vi "test_rig_main.vi"(10 "Pressure Controls":T1={"Atm Press"=0.0, "Des P drop"=0.0, "Phi"=0.0, "PID gains"={"proportional gain (Kc)"=3.0, "integral time (Ti, min)"=0.0003, "derivative time (Td, min)"=-0.0001}, "output range"={"output high"=400.0, "output low"=0.0003}, "Run Mode"=enum."Non pre-mixed"} {"output range"."output low" format="%.2f"; "output range"."output high" format="%.2f"; "PID gains"."derivative time (Td, min)" format="%.6f"; "PID gains"."integral time (Ti, min)" format="%.5f"; "PID gains"."proportional gain (Kc)" format="%.3f"; "Phi" scale=0.0..1.5; "Des P drop" scale=0.0..6.0}) -> (2 "Pressure Indicators":T3 {"Measured Pressure (psi abs)" scale=0.0..6.0})   [LabVIEW 2013]
doc: "This is the main VI for the test rig program. It allows the user to control fuel flow to burners, and move\nthe three-axis table."
uses:
  Controls/pressure_control_cluster.ctl
  Controls/run_mode_enum.ctl
  Controls/pressure_indicator_cluster.ctl
  Controls/enable_control_cluster.ctl
  Controls/manual_feed_control_cluster.ctl
  Controls/axis_indicator_cluster.ctl
  Controls/auto_feed_control_cluster.ctl
  <vilib>/MotionAssistant/MotionAssistant.llb/Move Constraints.ctl
  <vilib>/MotionAssistant/MotionAssistant.llb/Velocity Profile Type Enum.ctl
  <vilib>/MotionAssistant/MotionAssistant.llb/Straight Line Move Properties.ctl
  <vilib>/MotionAssistant/MotionAssistant.llb/Straight Line Dimension Enum.ctl
  <vilib>/MotionAssistant/MotionAssistant.llb/Straight Line Move Mode Enum.ctl
  <vilib>/MotionAssistant/MotionAssistant.llb/Coordinate Point.ctl
  <vilib>/MotionAssistant/MotionAssistant.llb/Profile Calculation Constraint.ctl
  <vilib>/MotionAssistant/MotionAssistant.llb/Array Constraints Spec Type Enum.ctl
  <vilib>/MotionAssistant/MotionAssistant.llb/Move Profile Enum.ctl
  Controls/PWM_data_cluster.ctl
  Controls/table_axis_enum.ctl
  Controls/PWM_state_enum.ctl
  <vilib>/DAQmx/read.llb/DAQmx Read (Analog DBL 1Chan 1Samp).vi
  <vilib>/DAQmx/write.llb/DAQmx Write (Digital Bool 1Line 1Point).vi
  <vilib>/MotionAssistant/MotionAssistant.llb/Open Straight Line Move Handle.vi
  <vilib>/MotionAssistant/MotionAssistant.llb/Close Straight Line Move Handle.vi
  <vilib>/DAQmx/miscellaneous.llb/DAQmx Fill In Error Info.vi
  <vilib>/MotionAssistant/MotionAssistant.llb/Set Straight Line Move Properties.vi
  <vilib>/MotionAssistant/MotionAssistant.llb/Get Straight Line Move Profile.vi
panel:
  in  "stop":bool
  in  "Control Tabs":enum32{"Master Control", "Table Control"}(tab)
  in  "Enabling Controls":T4 {"Number of Images" min=0 step=1}
  out "UV Image":T5(plugin-control)
  in  "Auto Fd. Ctrl.":T6 caption="Auto Feed Control"
  out "Axis Inds.":T7 caption="Axis Indicators"
  in  "Man. Fd. Ctrl.":T8 caption="Manual Feed Control"
  in  "Move Constraints":T9={"Velocity Profile Type"=enum."S Curve", "Max Velocity"=2.0, "Max Acceleration"=1.0, "Max Deceleration"=1.0, "Max Jerk"=2.0, "Initial Velocity"=0.0, "Final Velocity"=0.0} {"Final Velocity" format="%#.6g"; "Initial Velocity" format="%#.6g"; "Max Jerk" format="%#.6g"; "Max Deceleration" format="%#.6g"; "Max Acceleration" format="%#.6g"; "Max Velocity" format="%#.6g"}
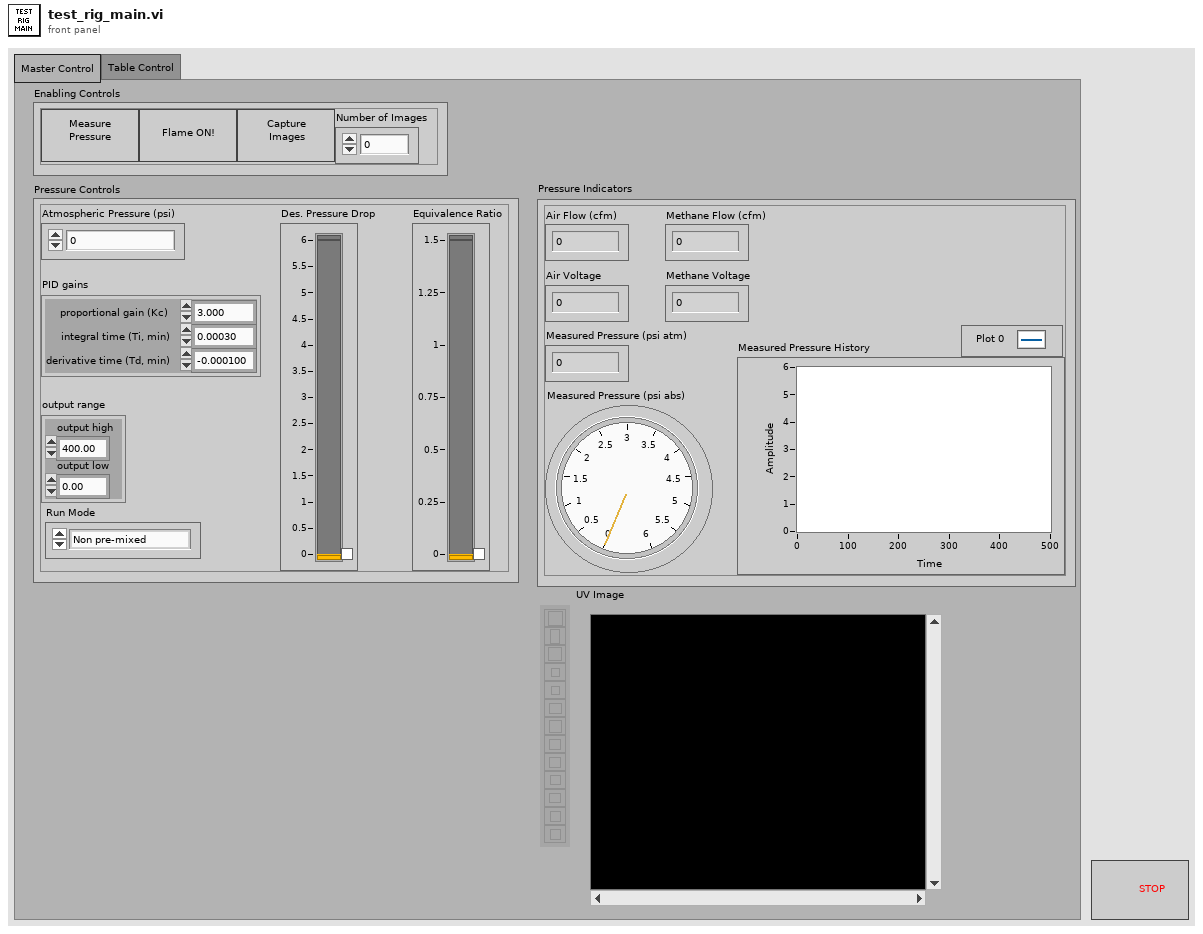
[diagram p1: front panel]
types:
  T1 = typedef "pressure_control_cluster.ctl" = cluster{"Atm Press":dbl, "Des P drop":dbl, "Phi":dbl, "PID gains":cluster{"proportional gain (Kc)":dbl, "integral time (Ti, min)":dbl, "derivative time (Td, min)":dbl}, "output range":cluster{"output high":dbl, "output low":dbl}, "Run Mode":T2}
  T2 = typedef "run_mode_enum.ctl" = enum16{"Non pre-mixed", "Pre-mixed"}
  T3 = typedef "pressure_indicator_cluster.ctl" = cluster{"Air Flow (cfm)":dbl, "Methane Flow (cfm)":dbl, "Air Voltage":dbl, "Methane Voltage":dbl, "Measured Pressure (psi atm)":dbl, "Measured Pressure (psi abs) ":dbl, "Measured Pressure History":dbl}
  T4 = typedef "enable_control_cluster.ctl" = cluster{"meas pressure":bool, "enable fuel":bool, "capture":bool, "Number of Images":i32}
  T5 = typedef "IMAQ Image.ctl" = refnum<image>
  T6 = typedef "auto_feed_control_cluster.ctl" = cluster{"Feed Rate (in/s)":dbl, "X Command (in)":dbl, "Y Command (in)":dbl, "Z Command (in)":dbl, "feed to pos":bool}
  T7 = typedef "axis_indicator_cluster.ctl" = cluster{"X Position (in)":dbl, "Y Position (in)":dbl, "Z Position (in)":dbl, "X Moving":bool, "Y Moving":bool, "Z Moving":bool, "Speed (in/s)":dbl}
  T8 = typedef "manual_feed_control_cluster.ctl" = cluster{"move -Y":bool, "move +Y":bool, "move -X":bool, "move +X":bool, "move +Z":bool, "move -Z":bool}
  T9 = typedef "Move Constraints.ctl" = cluster{"Velocity Profile Type":T10, "Max Velocity":dbl, "Max Acceleration":dbl, "Max Deceleration":dbl, "Max Jerk":dbl, "Initial Velocity":dbl, "Final Velocity":dbl}
  T10 = typedef "Velocity Profile Type Enum.ctl" = enum32{"Trapezoidal", "S Curve"}
  T11 = typedef "Straight Line Move Properties.ctl" = cluster{"Dimension":T12, "Move Mode":T13, "Position Mode - End Point":T14, "Velocity Mode - Travel Time (sec)":dbl}
  T12 = typedef "Straight Line Dimension Enum.ctl" = enum16{"1-Dimension", "2-Dimension", "3-Dimension"}
  T13 = typedef "Straight Line Move Mode Enum.ctl" = enum32{" Position Mode", "Velocity Mode"}
  T14 = typedef "Coordinate Point.ctl" = cluster{"X":dbl, "Y":dbl, "Z":dbl}
  T15 = cluster{"Straight Line Move Properties":T11, "Start Point":T14}
  T16 = typedef "Straight Line Move Handle.ctl" = cluster{"Straight Line Move Enum":T17, "Move Handle":i32}
  T17 = typedef "Straight Line Move Enum.ctl" = enum16{"Straight Line Move"}
  T18 = typedef "PWM_data_cluster.ctl" = cluster{"frequency":dbl, "Duty Cycle (%)":dbl, "Axis Enum":T19, "Function Enum":T20}
  T19 = typedef "table_axis_enum.ctl" = enum16{"X-axis", "Y-axis", "Z-axis", "W-axis"}
  T20 = typedef "PWM_state_enum.ctl" = enum16{"Initialize", "SetAxisSpeed", "StopAxis", "StopAll", "Shutdown"}
  T21 = typedef "Move Profile Enum.ctl" = enum16{"Velocity Profile", "Acceleration Profile", "Position Profile"}
  T22 = typedef "Profile Calculation Constraint.ctl" = cluster{"Constraint Type":T23, "Constraint Value":dbl}
  T23 = typedef "Array Constraints Spec Type Enum.ctl" = enum16{"Array Size", "Sampling Time"}
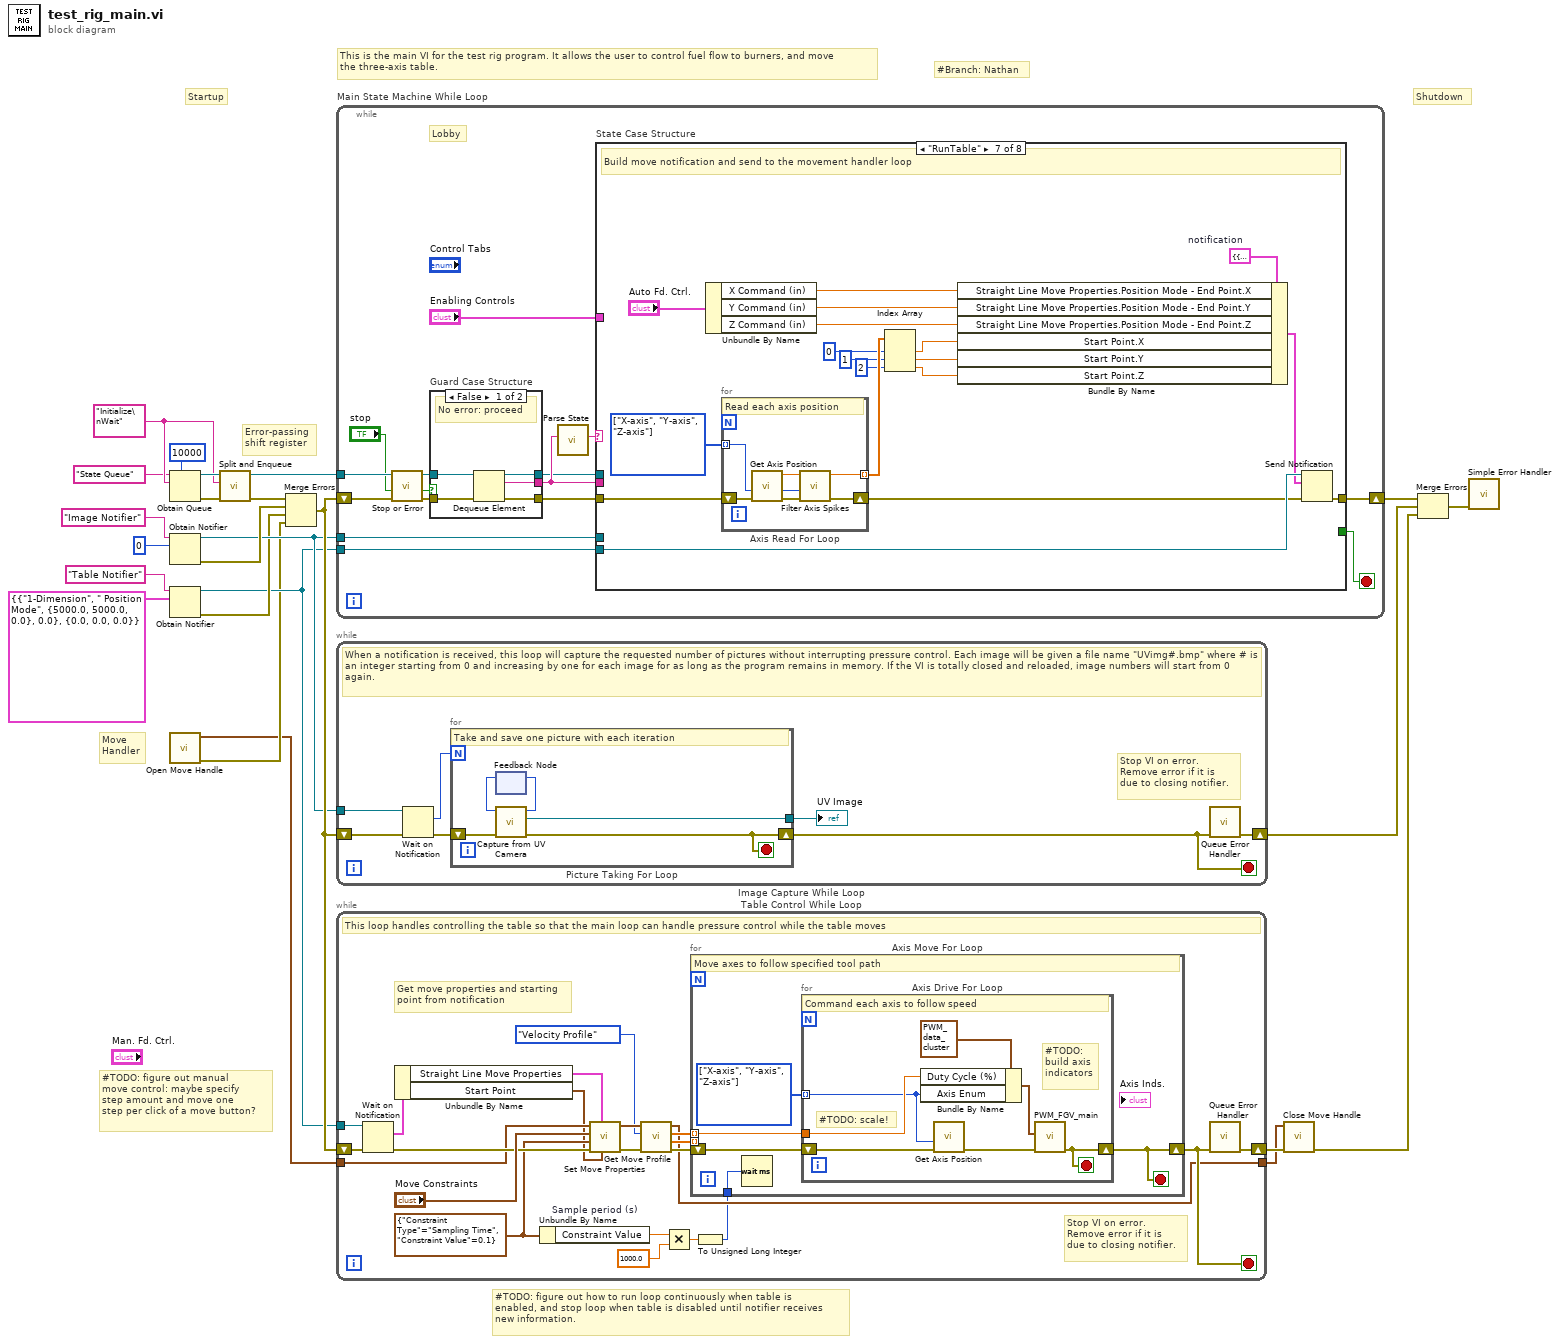
[diagram p0: block diagram]
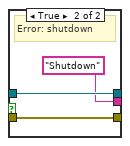
[diagram p2: hidden frame]
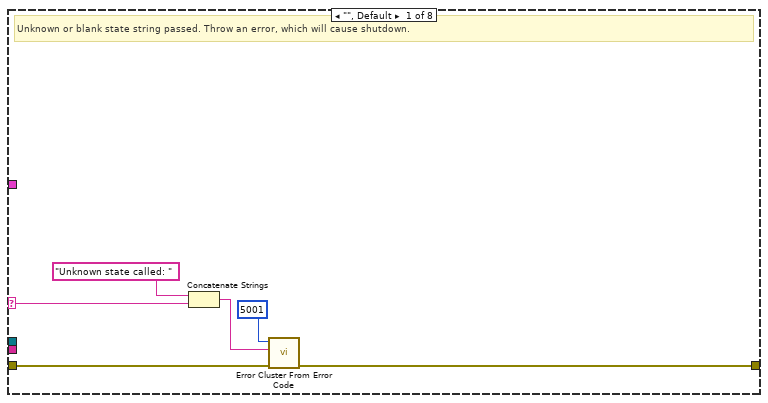
[diagram p3: hidden frame]
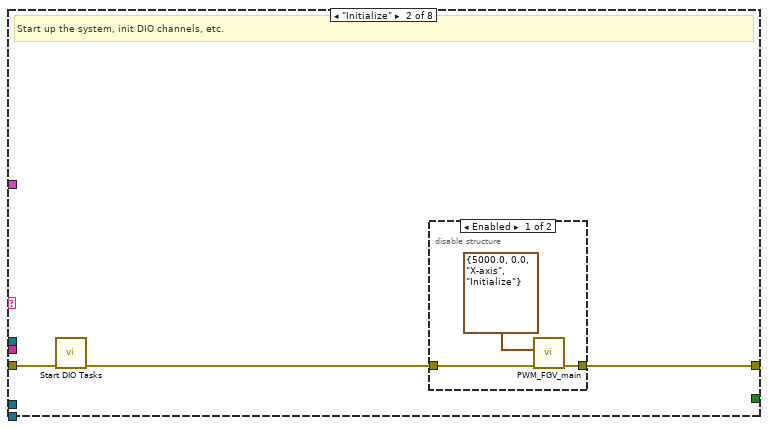
[diagram p4: hidden frame]
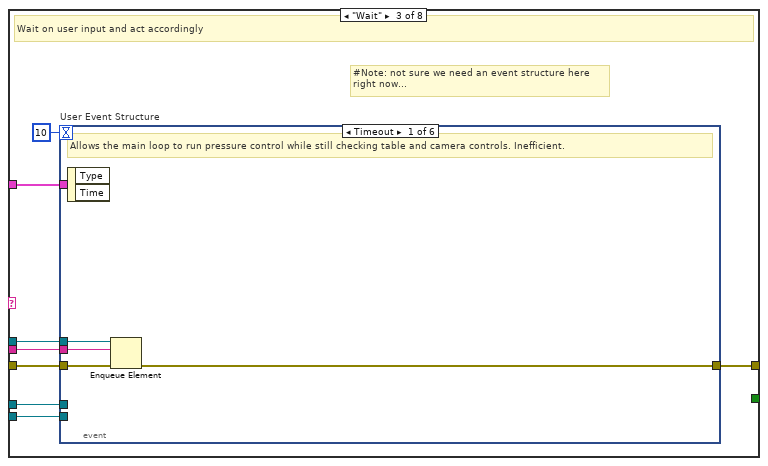
[diagram p6: hidden frame]
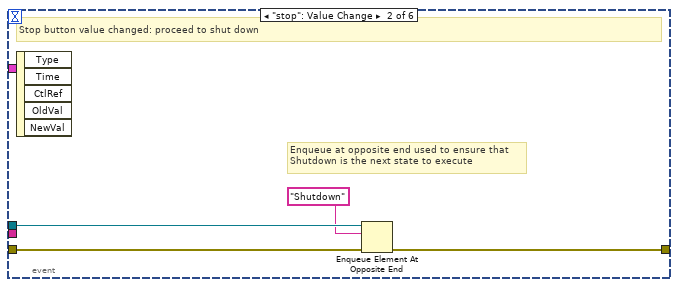
[diagram p7: hidden frame]
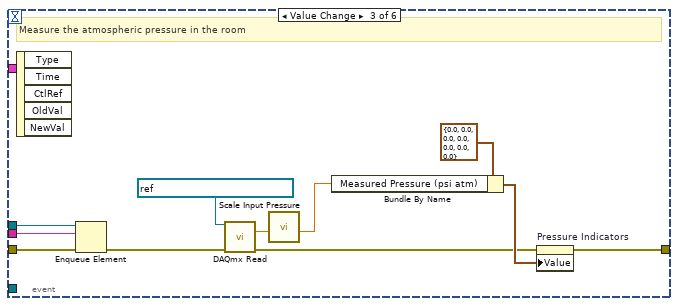
[diagram p8: hidden frame]
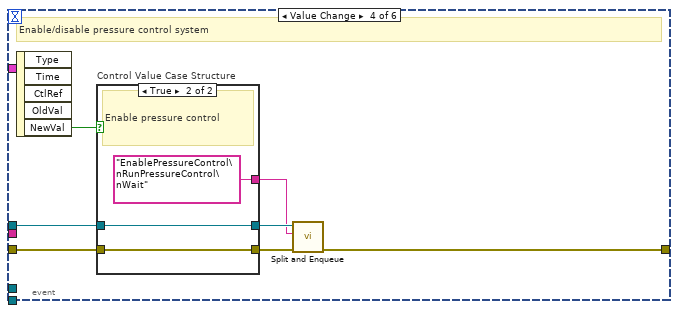
[diagram p9: hidden frame]
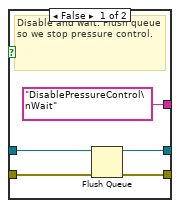
[diagram p10: hidden frame]
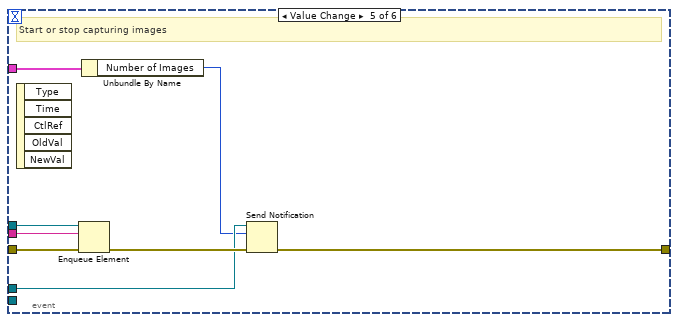
[diagram p11: hidden frame]
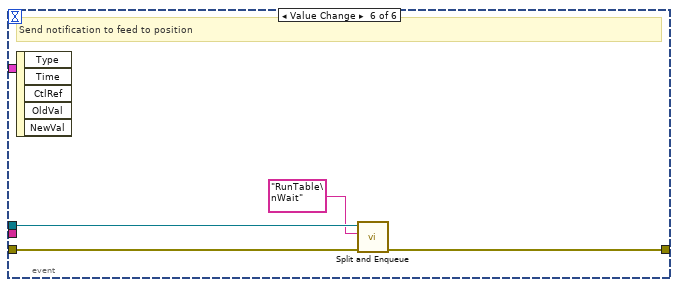
[diagram p12: hidden frame]
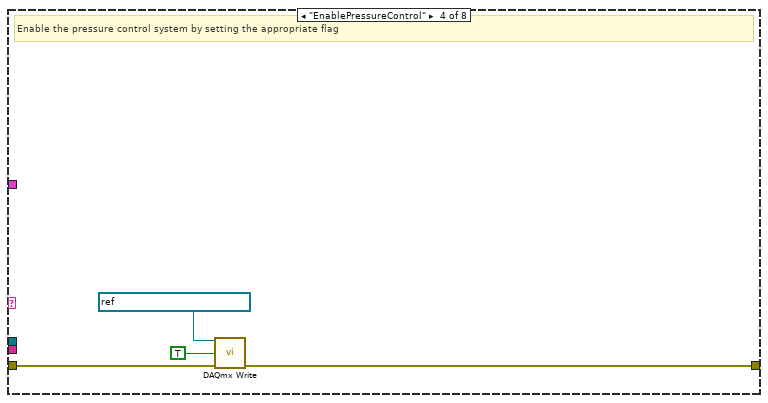
[diagram p13: hidden frame]
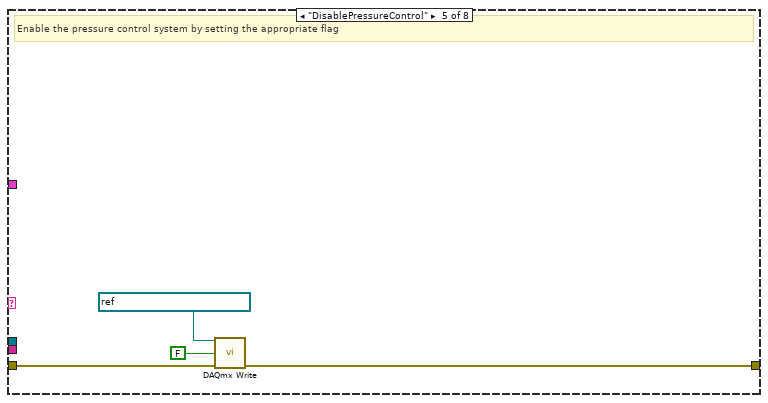
[diagram p14: hidden frame]
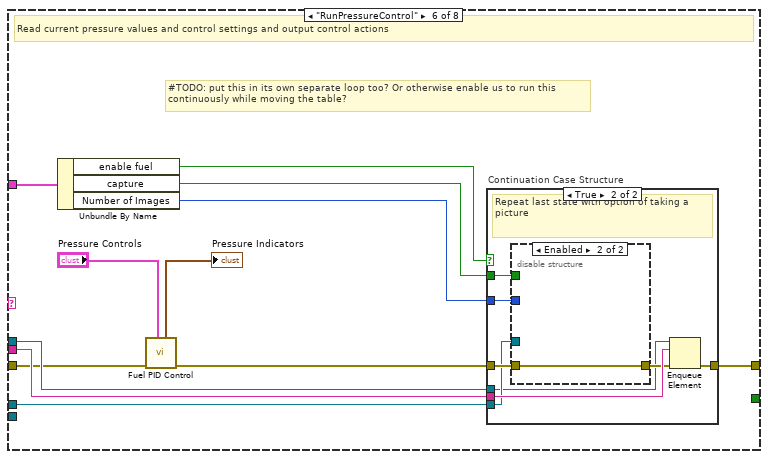
[diagram p15: hidden frame]
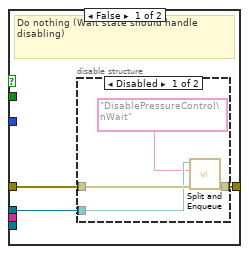
[diagram p16: hidden frame]
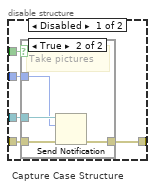
[diagram p18: hidden frame]
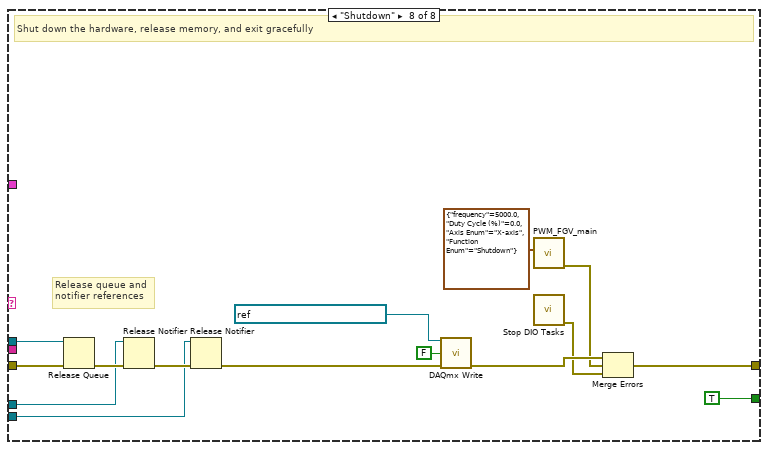
[diagram p20: hidden frame]
diagram:
  w20 = "Initialize\nWait"
  # "#Branch: Nathan"
  # "#TODO: figure out manual\nmove control: maybe specify\nstep amount and move one\nstep per click of a move button?"
  # "Move\nHandler"
  # "#TODO: figure out how to run loop continuously when table is\nenabled, and stop loop when table is disabled until notifier receives\nnew information."
  # "Shutdown"
  # "Startup"
  # "Error-passing\nshift register"
  # "This is the main VI for the test rig program. It allows the user to control fuel flow to burners, and move\nthe three-axis table."
  n1 = Obtain Queue(max queue size (-1, unlimited)=10000, name (unnamed)="State Queue", element data type=w20) -> (queue out=w22:refnum<queue>, error out=w23:errorcluster)  [unwired: 2 in, 1 out]
  n2 = Obtain Notifier(name (unnamed)="Image Notifier", notification data type=0) -> (notifier out=w10:refnum<notifier>, error out=w13:errorcluster)  [unwired: 2 in, 1 out]
  n3 = Obtain Notifier(name (unnamed)="Table Notifier", notification data type=T15 {"Straight Line Move Properties"={"Dimension"=enum."1-Dimension", "Move Mode"=enum." Position Mode", "Position Mode - End Point"={"X"=5000.0, "Y"=5000.0, "Z"=0.0}, "Velocity Mode - Travel Time (sec)"=0.0}, "Start Point"={"X"=0.0, "Y"=0.0, "Z"=0.0}}) -> (notifier out=w7:refnum<notifier>, error out=w9:errorcluster)  [unwired: 2 in, 1 out]
  n4 = call-poly <vilib>:"Open Move Handle.vi"() -> ("error out"=w6:errorcluster, "Straight Line Move Handle"=w5:T16)  [unwired: 9 in]
  n5 = call "Split and Enqueue.vi"("error in (no error)"=w23, "Input String"=w20, "queue in"=w22) -> ("error out"=w14:errorcluster, "queue out"=w21:refnum<queue>)  [unwired: 7 in]
  n6 = Merge Errors(w14, w13, w9, w6) -> (w11:errorcluster)
  n7 = while "Main State Machine While Loop" {
    tunnel: w21 -> [w38]
    shift-right: [w29] -> w12
    shift-left: w11 -> [w37]
    tunnel: w10 -> [w26]
    tunnel: w7 -> [w25]
    stop <- w28 stop-if-true
    # "Lobby"
    n8 = call "Stop or Error.vi"("Error In"=w37, "Stop Button"="stop") -> ("Error Out"=w36:errorcluster, "Stop or Error?"=w35:bool)  [unwired: 8 in]
    n9 = case "Guard Case Structure" shown="False" w35 {
      tunnel: w38 -> [w41 w45]
      tunnel: w36 -> [w43 w46]
      tunnel: [w42 w46] -> w30
      tunnel: [w40 w45] -> w31
      tunnel: [w39 "Shutdown"] -> w33
      frame False {
        # "No error: proceed"
        n10 = Dequeue Element(queue=w41, error in (no error)=w43) -> (queue out=w40:refnum<queue>, element=w39:string, error out=w42:errorcluster)  [unwired: 1 in, 1 out]
      }
      frame True {
        # "Error: shutdown"
      }
    }
    n11 = call "Parse State.vi"("String with Args"=w33) -> ("State"=w32:string)  [unwired: 10 in]
    n12 = case "State Case Structure" shown="\"RunTable\"" w32 {
      selector: w32 -> [w49 _ _ _ _ _ _ _]
      tunnel: w33 -> [_ _ w64 _ _ w131 _ _]
      tunnel: w31 -> [_ _ w65 _ _ w132 _ w199]
      tunnel: w30 -> [w52 w55 w67 w117 w119 w128 w178 w200]
      tunnel: [w51 w54 w66 w116 w118 w133 w173 w197] -> w29
      tunnel: [_ _ _ _ _ _ _ TRUE] -> w28
      tunnel: "Enabling Controls" -> [_ _ w63 _ _ w130 _ _]
      tunnel: w26 -> [_ _ w62 _ _ w123 _ w189]
      tunnel: w25 -> [_ _ w61 _ _ _ w172 w186]
      frame "", Default {
        # "Unknown or blank state string passed. Throw an error, which will cause shutdown."
        n13 = Concatenate Strings("Unknown state called: " ("string"), w49) -> (w48:string)
        n14 = call <vilib>:"Error Cluster From Error Code.vi"("error in (no error)"=w52, "error message (\"\")"=w48, "error code (0)"=5001) -> ("error out"=w51:errorcluster)  [unwired: 6 in]
      }
      frame "Initialize" {
        # "Start up the system, init DIO channels, etc."
        n15 = call "Start DIO Tasks.vi"("error in (no error)"=w55) -> ("error out"=w53:errorcluster)  [unwired: 10 in]
        n16 = disable-structure shown="Enabled" {
          disable-tunnel: w53 -> [w56 w59]
          disable-tunnel: [w58 w59] -> w54
          frame Enabled {
            n17 = call "PWM_FGV_main.vi"("Error In"=w56, "PWM FGV Data"=T18 {"frequency"=5000.0, "Duty Cycle (%)"=0.0, "Axis Enum"=enum."X-axis", "Function Enum"=enum."Initialize"}) -> ("Error Out"=w58:errorcluster)  [unwired: 9 in]
          }
          frame Disabled {
          }
        }
      }
      frame "Wait" {
        # "#Note: not sure we need an event structure here\nright now..."
        # "Wait on user input and act accordingly"
        n18 = event "User Event Structure" shown="[0] Timeout" {
          selector: _ -> [_ _ _ _ _ _]
          dyn-events: _ -> [_ _ _ _ _ _]
          timeout: 10 -> [_ _ _ _ _ _]
          tunnel: w67 -> [w71 w75 w86 w92 w108 w112]
          tunnel: [w70 w74 w79 w89 w102 w113] -> w66
          tunnel: w65 -> [w69 w73 w83 w91 w107 w111]
          tunnel: w64 -> [w68 _ w76 _ w106 _]
          tunnel: w63 -> [_ _ _ _ w109 _]
          tunnel: w62 -> [_ _ _ _ w104 _]
          tunnel: w61 -> [_ _ _ _ _ _]
          event Timeout {
            # "Allows the main loop to run pressure control while still checking table and camera controls. Inefficient."
            n19 = event-data() -> ()  [unwired: 1 in, 2 out]
            n20 = Enqueue Element(queue=w69, element=w68, error in (no error)=w71) -> (error out=w70:errorcluster)  [unwired: 1 in, 2 out]
          }
          event "stop": Value Change {
            # "Enqueue at opposite end used to ensure that\nShutdown is the next state to execute"
            # "Stop button value changed: proceed to shut down"
            n21 = event-data() -> ()  [unwired: 1 in, 5 out]
            n22 = Enqueue Element At Opposite End(queue=w73, element="Shutdown", error in (no error)=w75) -> (error out=w74:errorcluster)  [unwired: 1 in, 2 out]
          }
          event Value Change {
            # "Measure the atmospheric pressure in the room"
            n23 = event-data() -> ()  [unwired: 1 in, 5 out]
            n24 = Enqueue Element(queue=w83, element=w76, error in (no error)=w86) -> (error out=w84:errorcluster)  [unwired: 1 in, 2 out]
            n25 = call-poly <vilib>:"DAQmx Read.vi"("task/channels in"=refnum<k21> "PressureVoltageIn_S3AI8", "error in"=w84) -> ("data"=w82:dbl, "error out"=w77:errorcluster)  [unwired: 11 in, 1 out]
            n26 = call "Scale Input Pressure.vi"("Pressure (V)"=w82) -> ("Pressure (psi atm)"=w80:dbl)  [unwired: 10 in]
            n27 = Bundle By Name(cluster=T3 {"Air Flow (cfm)"=0.0, "Methane Flow (cfm)"=0.0, "Air Voltage"=0.0, "Methane Voltage"=0.0, "Measured Pressure (psi atm)"=0.0, "Measured Pressure (psi abs) "=0.0, "Measured Pressure History"=0.0} ("Pressure Indicators 2"), "Measured Pressure (psi atm)"=w80) -> (w78:T3)
            n28 = property on="Pressure Indicators" class="Clust (strict)"(error in=w77, "Value"=w78) -> (error out=w79:errorcluster)  [unwired: 1 in, 1 out]
          }
          event Value Change {
            # "Enable/disable pressure control system"
            n29 = event-data() -> ("NewVal"=w93:bool)  [unwired: 1 in, 4 out]
            n30 = case "Control Value Case Structure" shown="True" w93 {
              tunnel: w92 -> [w98 w101]
              tunnel: [w96 w101] -> w90
              tunnel: w91 -> [w97 w99]
              tunnel: [w95 w99] -> w88
              tunnel: ["DisablePressureControl\nWait" ("Input String") "EnablePressureControl\nRunPressureControl\nWait" ("Input String")] -> w87
              frame False {
                # "Disable and wait. Flush queue so we stop pressure control."
                n31 = Flush Queue(queue=w97, error in (no error)=w98) -> (queue out=w95:refnum<queue>, error out=w96:errorcluster)  [unwired: 1 out]
              }
              frame True {
                # "Enable pressure control"
              }
            }
            n32 = call "Split and Enqueue.vi"("error in (no error)"=w90, "Input String"=w87, "queue in"=w88) -> ("error out"=w89:errorcluster)  [unwired: 7 in, 1 out]
          }
          event Value Change {
            # "Start or stop capturing images"
            n33 = event-data() -> ()  [unwired: 1 in, 5 out]
            n34 = Enqueue Element(queue=w107, element=w106, error in (no error)=w108) -> (error out=w105:errorcluster)  [unwired: 1 in, 2 out]
            n35 = Unbundle By Name(w109) -> ("Number of Images"=w103:i32)
            n36 = Send Notification(notification=w103, notifier=w104, error in (no error)=w105) -> (error out=w102:errorcluster)  [unwired: 1 out]
          }
          event Value Change {
            # "Send notification to feed to position"
            n37 = event-data() -> ()  [unwired: 1 in, 5 out]
            n38 = call "Split and Enqueue.vi"("error in (no error)"=w112, "Input String"="RunTable\nWait", "queue in"=w111) -> ("error out"=w113:errorcluster)  [unwired: 7 in, 1 out]
          }
        }
      }
      frame "EnablePressureControl" {
        # "Enable the pressure control system by setting the appropriate flag"
        n39 = call-poly <vilib>:"DAQmx Write.vi"("task/channels in"=refnum<k21> "RemoteEnable_S3P00L0", "data"=TRUE, "error in"=w117) -> ("error out"=w116:errorcluster)  [unwired: 10 in, 2 out]
      }
      frame "DisablePressureControl" {
        # "Enable the pressure control system by setting the appropriate flag"
        n40 = call-poly <vilib>:"DAQmx Write.vi"("task/channels in"=refnum<k21> "RemoteEnable_S3P00L0", "data"=FALSE, "error in"=w119) -> ("error out"=w118:errorcluster)  [unwired: 10 in, 2 out]
      }
      frame "RunPressureControl" {
        # "#TODO: put this in its own separate loop too? Or otherwise enable us to run this\ncontinuously while moving the table?"
        # "Read current pressure values and control settings and output control actions"
        n41 = Unbundle By Name(w130) -> ("enable fuel"=w129:bool, "capture"=w125:bool, "Number of Images"=w122:i32)
        n42 = call "Fuel PID Control.vi"("Pressure Controls"="Pressure Controls", "Error In"=w128) -> ("Error Out"=w127:errorcluster, "Pressure Indicators"=→"Pressure Indicators":T3)  [unwired: 8 in]
        n43 = case "Continuation Case Structure" shown="True" w129 {
          tunnel: w127 -> [w135 w147]
          tunnel: [w136 w149] -> w133
          tunnel: w132 -> [w134 w142]
          tunnel: w131 -> [_ w148]
          tunnel: w125 -> [_ w146]
          tunnel: w123 -> [_ w144]
          tunnel: w122 -> [_ w143]
          frame False {
            # "Do nothing (Wait state should handle disabling)"
            n44 = disable-structure shown="Disabled" {
              disable-tunnel: [w140 w141] -> w136
              disable-tunnel: w135 -> [w139 w141]
              disable-tunnel: w134 -> [w138 _]
              frame Disabled {
                n45 = call "Split and Enqueue.vi"("error in (no error)"=w139, "Input String"="DisablePressureControl\nWait", "queue in"=w138) -> ("error out"=w140:errorcluster)  [unwired: 7 in, 1 out]
              }
              frame Enabled {
              }
            }
          }
          frame True {
            # "Repeat last state with option of taking a picture"
            n46 = disable-structure shown="Enabled" {
              disable-tunnel: w147 -> [w154 w160]
              disable-tunnel: w146 -> [w153 _]
              disable-tunnel: [w152 w160] -> w145
              disable-tunnel: w144 -> [w151 _]
              disable-tunnel: w143 -> [w150 _]
              frame Disabled {
                n47 = case "Capture Case Structure" shown="True" w153 {
                  tunnel: w154 -> [w155 w158]
                  tunnel: [w155 w159] -> w152
                  tunnel: w151 -> [_ w157]
                  tunnel: w150 -> [_ w156]
                  frame False {
                    # "Pass through"
                  }
                  frame True {
                    # "Take pictures"
                    n48 = Send Notification(notification=w156, notifier=w157, error in (no error)=w158) -> (error out=w159:errorcluster)  [unwired: 1 out]
                  }
                }
              }
              frame Enabled {
              }
            }
            n49 = Enqueue Element(queue=w142, element=w148, error in (no error)=w145) -> (error out=w149:errorcluster)  [unwired: 1 in, 2 out]
          }
        }
      }
      frame "RunTable" {
        w169 = T19[] [enum."X-axis", enum."Y-axis", enum."Z-axis"] items=["X-axis", "Y-axis", "Z-axis", "W-axis"]
        w170 = T15 {"Straight Line Move Properties"={"Dimension"=enum."1-Dimension", "Move Mode"=enum." Position Mode", "Position Mode - End Point"={"X"=0.0, "Y"=0.0, "Z"=0.0}, "Velocity Mode - Travel Time (sec)"=0.0}, "Start Point"={"X"=0.0, "Y"=0.0, "Z"=0.0}}  # notification
        # "Build move notification and send to the movement handler loop"
        n50 = Unbundle By Name("Auto Fd. Ctrl.") -> ("X Command (in)"=w176:dbl, "Y Command (in)"=w175:dbl, "Z Command (in)"=w174:dbl)
        n51 = for "Axis Read For Loop" {
          shift-right: [w182] -> w171
          shift-left: w178 -> [w185]
          tunnel: w169 -> [w184] mode=indexing
          tunnel: [w179] -> w167 mode=indexing
          # "Read each axis position"
          n52 = call "Get Axis Position.vi"("Error In"=w185, "Axis Enum"=w184) -> ("Error Out"=w183:errorcluster, "Axis Enum Out"=w180:T19, "Axis Inches"=w181:dbl)  [unwired: 6 in, 1 out]
          n53 = call "Filter Axis Spikes.vi"("Error In"=w183, "Axis Enum"=w180, "Current Reading"=w181) -> ("Error Out"=w182:errorcluster, "Filtered Reading"=w179:dbl)  [unwired: 5 in, 2 out]
        }
        n54 = Index Array(array=w167, index #1=0 ("index"), index #2=1 ("index"), index #3=2 ("index")) -> (element #1=w163:dbl, element #2=w162:dbl, element #3=w161:dbl)
        n55 = Bundle By Name(cluster=w170, "Straight Line Move Properties.Position Mode - End Point.X"=w176, "Straight Line Move Properties.Position Mode - End Point.Y"=w175, "Straight Line Move Properties.Position Mode - End Point.Z"=w174, "Start Point.X"=w163, "Start Point.Y"=w162, "Start Point.Z"=w161) -> (w168:T15)
        n56 = Send Notification(notification=w168, notifier=w172, error in (no error)=w171) -> (error out=w173:errorcluster)  [unwired: 1 out]
      }
      frame "Shutdown" {
        # "Release queue and\nnotifier references"
        # "Shut down the hardware, release memory, and exit gracefully"
        n57 = Release Queue(queue=w199, error in (no error)=w200) -> (error out=w190:errorcluster)  [unwired: 1 in, 2 out]
        n58 = Release Notifier(notifier=w189, error in (no error)=w190) -> (error out=w188:errorcluster)  [unwired: 1 in, 2 out]
        n59 = Release Notifier(notifier=w186, error in (no error)=w188) -> (error out=w187:errorcluster)  [unwired: 1 in, 2 out]
        n60 = call-poly <vilib>:"DAQmx Write.vi"("task/channels in"=refnum<k21> "RemoteEnable_S3P00L0", "data"=FALSE, "error in"=w187) -> ("error out"=w194:errorcluster)  [unwired: 10 in, 2 out]
        n61 = call "PWM_FGV_main.vi"("PWM FGV Data"=T18 {"frequency"=5000.0, "Duty Cycle (%)"=0.0, "Axis Enum"=enum."X-axis", "Function Enum"=enum."Shutdown"}) -> ("Error Out"=w193:errorcluster)  [unwired: 10 in]
        n62 = call "Stop DIO Tasks.vi"() -> ("error out"=w191:errorcluster)  [unwired: 11 in]
        n63 = Merge Errors(w194, w193, w191) -> (w197:errorcluster)
      }
    }
  }
  n64 = while "Image Capture While Loop" {
    shift-right: [w202] -> w19
    shift-left: w11 -> [w207]
    tunnel: w10 -> [w206]
    stop <- w201 stop-if-true
    # "Stop VI on error.\nRemove error if it is\ndue to closing notifier."
    # "When a notification is received, this loop will capture the requested number of pictures without interrupting pressure control. Each image will be given a file name \"UVimg#.bmp\" where # is an integer starting from 0 and increasing by one for each image for as long as the program remains in memory. If the VI is totally closed and reloaded, image numbers will start from 0 again."
    n65 = Wait on Notification(notifier=w206, error in (no error)=w207) -> (notification=w203:i32, error out=w204:errorcluster)  [unwired: 2 in, 2 out]
    n66 = for "Picture Taking For Loop" {
      N: w203 -> [_]
      tunnel: [w210] -> w205
      shift-right: [w211] -> w201
      shift-left: w204 -> [w212]
      stop <- w211 stop-if-true
      # "Take and save one picture with each iteration"
      n67 = feedback #1() -> (w208:i32)  [unwired: 1 in]
      n68 = call "Capture from UV Camera.vi"("error in"=w212, "Image number in"=w208) -> ("error out"=w211:errorcluster, "Image Out"=w210:T5, "Image number out"=w209:i32)  [unwired: 7 in]
      n69 = feedback-in #1(w209) -> ()
    }
    "UV Image" <- w205
    n70 = call "Queue Error Handler.vi"("Error In"=w201) -> ("Error Out"=w202:errorcluster)  [unwired: 10 in]
  }
  n71 = while "Table Control While Loop" {
    shift-right: [w234] -> w4
    shift-left: w11 -> [w233]
    tunnel: w7 -> [w232]
    tunnel: w5 -> [w224]
    tunnel: [w222] -> w2
    stop <- w223 stop-if-true
    w220 = T22 {"Constraint Type"=enum."Sampling Time", "Constraint Value"=0.1} ("Profile Calculation Constraint")
    # "Get move properties and starting\npoint from notification"
    # "Stop VI on error.\nRemove error if it is\ndue to closing notifier."
    # "This loop handles controlling the table so that the main loop can handle pressure control while the table moves"
    n72 = Wait on Notification(notifier=w232, error in (no error)=w233) -> (notification=w215:T15, error out=w225:errorcluster)  [unwired: 2 in, 2 out]
    n73 = Unbundle By Name(w215) -> ("Straight Line Move Properties"=w214:T11, "Start Point"=w213:T14)
    n74 = Unbundle By Name "Sample period (s)"(w220) -> ("Constraint Value"=w217:dbl)
    n75 = call-poly <vilib>:"Set Move Properties.vi"("Start Point"=w213, "Straight Line Move Properties"=w214, "error in"=w225, "Profile Calculation Constraint"=w220, "Move Constraints"="Move Constraints", "Straight Line Move Handle In"=w224) -> ("error out"=w231:errorcluster, "Straight Line Move Handle Out"=w230:T16)  [unwired: 3 in]
    n76 = call-poly <vilib>:"Get Move Profile.vi"("error in"=w231, "Profile Type"=Move_Profile_Enum."Velocity Profile", "Straight Line Move Handle In"=w230) -> ("error out"=w229:errorcluster, "Time Indices"=w227:dbl[], "Profile"=w228:dbl[], "Straight Line Move Handle Out"=w222:T16)  [unwired: 3 in, 1 out]
    n77 = Multiply(x=w217, y=1000.0) -> (x*y=w218:dbl)
    n78 = To Unsigned Long Integer(number=w218) -> (unsigned 32bit integer=w219:u32)
    n79 = for "Axis Move For Loop" {
      shift-right: [w237] -> w223
      shift-left: w229 -> [w239]
      tunnel: w228 -> [w236] mode=indexing
      tunnel: w227 -> [_] mode=indexing
      tunnel: w219 -> [w238]
      stop <- w237 stop-if-true
      w235 = T19[] [enum."X-axis", enum."Y-axis", enum."Z-axis"] items=["X-axis", "Y-axis", "Z-axis", "W-axis"]
      # "Move axes to follow specified tool path"
      n80 = Wait (ms)(milliseconds to wait=w238) -> ()  [unwired: 1 out]
      n81 = for "Axis Drive For Loop" {
        tunnel: w236 -> [w244]
        tunnel: w235 -> [w240] mode=indexing
        shift-right: [w241] -> w237
        shift-left: w239 -> [w243]
        stop <- w241 stop-if-true
        # "#TODO:\nbuild axis\nindicators"
        # "#TODO: scale!"
        # "Command each axis to follow speed"
        n82 = Bundle By Name(cluster=T18 {"frequency"=5000.0, "Duty Cycle (%)"=0.0, "Axis Enum"=enum."X-axis", "Function Enum"=enum."Shutdown"} ("PWM FGV Data"), "Duty Cycle (%)"=w244, "Axis Enum"=w240) -> (w245:T18)
        n83 = call "Get Axis Position.vi"("Error In"=w243, "Axis Enum"=w240) -> ("Error Out"=w242:errorcluster)  [unwired: 6 in, 3 out]
        n84 = call "PWM_FGV_main.vi"("Error In"=w242, "PWM FGV Data"=w245) -> ("Error Out"=w241:errorcluster)  [unwired: 9 in]
      }
    }
    n85 = call "Queue Error Handler.vi"("Error In"=w223) -> ("Error Out"=w234:errorcluster)  [unwired: 10 in]
  }
  n86 = call-poly <vilib>:"Close Move Handle.vi"("error in"=w4, "Straight Line Move Handle"=w2) -> ("error out"=w3:errorcluster)  [unwired: 8 in]
  n87 = Merge Errors(w12, w19, w3) -> (w18:errorcluster)
  n88 = call <vilib>:"Simple Error Handler.vi"("error in (no error)"=w18) -> ()  [unwired: 4 in, 5 out]
